vi "VoltageScan_Old.vi"() -> ()   [LabVIEW 2016]
uses:
  <instrlib>/Keithley 24XX/Public/Data/Read (Statistical).vi
  <instrlib>/Keithley 24XX/Public/Data/Read (Single Point).vi
  <instrlib>/Keithley 24XX/Keithley 24XX.lvlib
  <instrlib>/Agilent 428X Series/Agilent 428X Series.lvlib
panel:
  out "error out":errorcluster
  in  "VISA resource name LCR":refnum<visa-resource-name>
  out "Data Status":bool=TRUE
  in  "Open (F:OFF)":bool
  in  "Short (F:OFF)":bool
  out "Primary Value":dbl format="%^.4e"
  out "Secondary Value":dbl format="%^.4e"
  in  "Imp Type (0: CPD)":u32(ring) items=["CPD", "CPQ", "CPG", "CPRP", "CSD", "CSQ", "CSRS", "LPQ", "LPD", "LPG", "LPRP", "LSD", "LSQ", "LSRS", "RX", "ZTD", "ZTR", "GB", "YTD", "YTR"]
  in  "Freq Value (Hz)(1.0 kHz)":dbl=1000.0 min=20.0 max=30000000.0 step=10.0 format="%.4e"
  in  "Voltage Level (V)(1.0V)":dbl=1.0 min=0.0 max=20.0 step=0.1 format="%.4f"
  in  "Measurement type":enum16{"IV", "CV", "Test"}(ring)
  out "Voltage":sgl
  out "Current*Resistance":sgl
  in  "Enable Voltage Auto Range (T:Enable)":bool=TRUE
  in  "Single measurement?":bool=TRUE
  in  "Statistical Operation (0: Mean)":u16(ring) items=["Mean", "Standard Deviation", "Maximum", "Minimum", "Peak to Peak"]
  in  "Sample Count (10)":i32=10
  in  "Source Mode  (0: Voltage)":u16(ring) items=["Voltage", "Current"]
  in  "Compliance  Level (uA)":dbl=0.1
  in  "Voltage":dbl=1.0
  in  "Voltage Manual Range (1.0)":dbl=1.0
  out "Resistance":sgl
  out "Current":sgl
  in  "Serial Configuration":T1={"Baud Rate"=9600, "Parity"=0, "Data Bits"=8, "Stop Bits"=10, "Flow Control"=0} {"Flow Control" items=["None", "XON/XOFF", "RTS/CTS", "XON/XOFF & RTS/CTS", "DTR/DSR", "XON/XOFF & DTR/DSR"]; "Stop Bits" items=["1.0"=10, "1.5"=15, "2.0"=20]; "Data Bits" items=["7"=7, "8"=8]; "Parity" items=["None", "Odd", "Even", "Mark", "Space"]; "Baud Rate" items=["300"=300, "600"=600, "1200"=1200, "2400"=2400, "4800"=4800, "9600"=9600, "19200"=19200]}
  in  "VISA resource name":refnum<visa-resource-name>
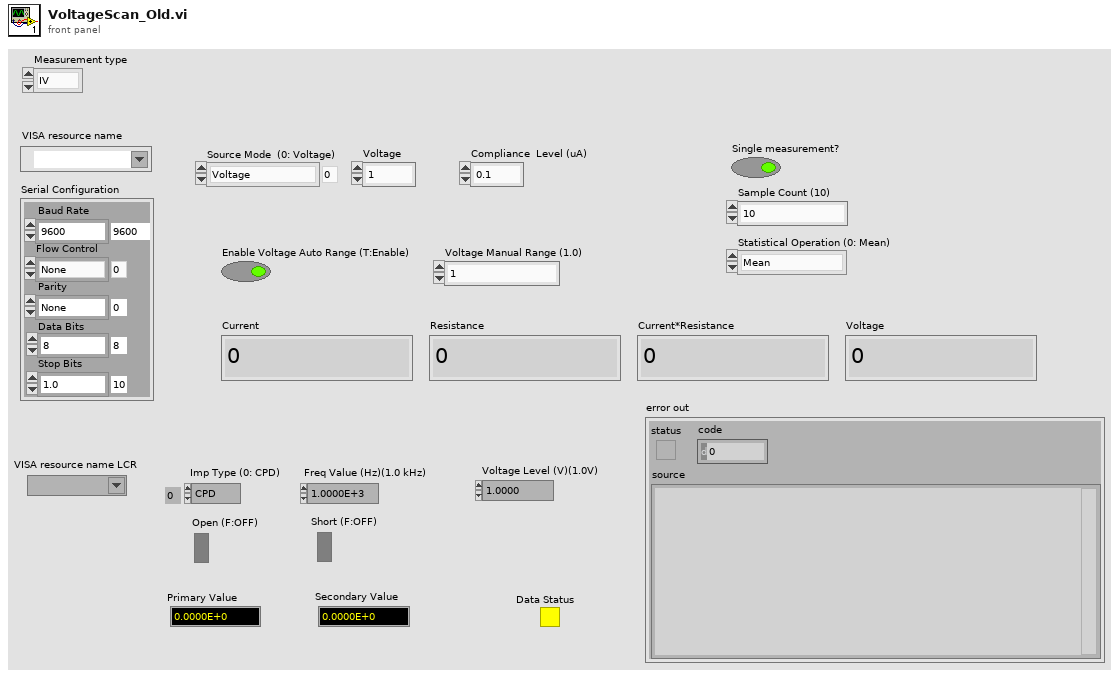
[diagram p1: front panel]
types:
  T1 = cluster{"Baud Rate":u32, "Parity":u16, "Data Bits":u16, "Stop Bits":u16, "Flow Control":u16}
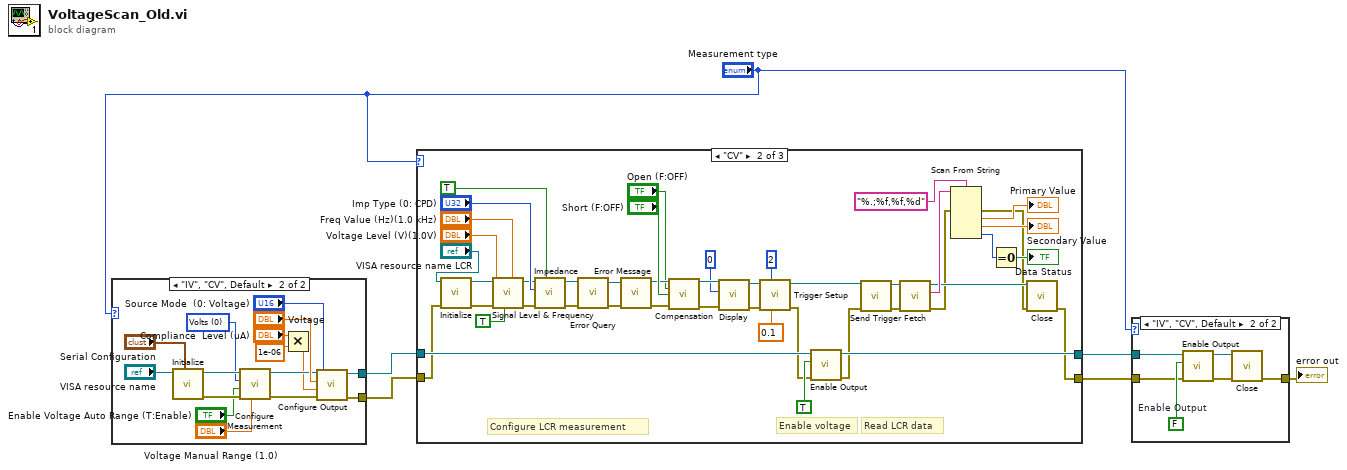
[diagram p0: block diagram]
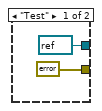
[diagram p3: hidden frame]
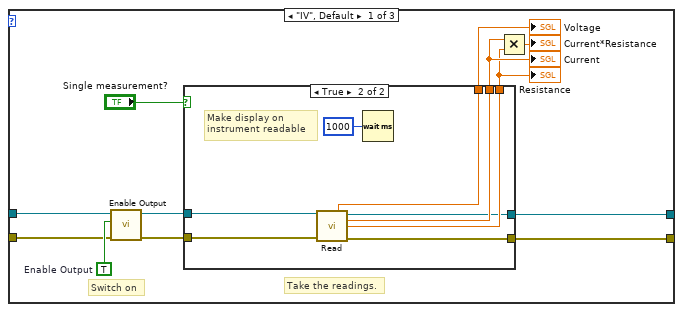
[diagram p4: hidden frame]
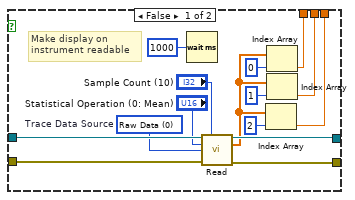
[diagram p5: hidden frame]
diagram:
  n1 = case shown="\"IV\", \"CV\", Default" "Measurement type" {
    tunnel: [errorcluster {"status"=FALSE, "code"=0, "source"=""} ("error out") w10] -> w4
    tunnel: [refnum<visa-resource-name> refnum ("VISA resource name out") w9] -> w3
    frame "Test" {
    }
    frame "IV", "CV", Default {
      w20 = u16 0 items=["Volts", "Current", "Resistance"] ("Function (0: Volts)")
      n2 = call <instrlib>:"Initialize.vi"("Serial Configuration"="Serial Configuration", "VISA resource name"="VISA resource name") -> ("error out"=w21:errorcluster, "VISA resource name out"=w22:refnum<visa-resource-name>)  [unwired: 8 in]
      n3 = call <instrlib>:"Configure Measurement.vi"("Manual Range (1.0)"="Voltage Manual Range (1.0)", "error in (no error)"=w21, "Enable Auto Range (T:Enable)"="Enable Voltage Auto Range (T:Enable)", "Function (0: Volts)"=w20, "VISA resource name"=w22) -> ("error out"=w15:errorcluster, "VISA resource name out"=w16:refnum<visa-resource-name>)  [unwired: 5 in]
      n4 = Multiply(x="Compliance  Level (uA)", y=1e-06) -> (x*y=w12:dbl)
      n5 = call <instrlib>:"Configure Output.vi"("Source Mode  (0: Voltage)"="Source Mode  (0: Voltage)", "error in (no error)"=w15, "Compliance  Level (0.1)"=w12, "Output Level (0)"="Voltage", "VISA resource name"=w16) -> ("error out"=w10:errorcluster, "VISA resource name out"=w9:refnum<visa-resource-name>)  [unwired: 5 in]
    }
  }
  n6 = case shown="\"CV\"" "Measurement type" {
    tunnel: [w36 w63 w104] -> w6
    tunnel: [w35 w101 w105] -> w5
    tunnel: w4 -> [w27 w75 w104]
    tunnel: w3 -> [w28 w102 w105]
    frame "IV", Default {
      w29 = TRUE  # Enable Output
      # "Take the readings."
      # "Switch on"
      n7 = call <instrlib>:"Enable Output.vi"("error in (no error)"=w27, "Enable Output (T: Enable)"=w29, "VISA resource name"=w28) -> ("error out"=w25:errorcluster, "VISA resource name out"=w26:refnum<visa-resource-name>)  [unwired: 7 in]
      n8 = case shown="True" "Single measurement?" {
        tunnel: [w42 w59] -> w32
        tunnel: [w41 w58] -> w31
        tunnel: [w50 w57] -> w36
        tunnel: [w48 w56] -> w35
        tunnel: w25 -> [w51 w55]
        tunnel: w26 -> [w49 w54]
        tunnel: [w38 w53] -> w30
        frame False {
          w43 = u16 0 items=["Raw Data", "Math Data", "Limit Data"]  # Trace Data Source
          # "Make display on instrument readable"
          n9 = Wait (ms)(milliseconds to wait=u32 1000) -> ()  [unwired: 1 out]
          n10 = call-poly <instrlib>:"Read.vi"("VISA resource name"=w49, "Sample Count (2)"="Sample Count (10)", "Statistical Operation (0: Mean)"="Statistical Operation (0: Mean)", "Trace Data Source (0: Raw Data)"=w43, "error in (no error)"=w51) -> ("VISA resource name out"=w48:refnum<visa-resource-name>, "Statistical Operation Results"=w39:dbl[], "error out"=w50:errorcluster)  [unwired: 8 in]
          n11 = Index Array(array=w39, index=2) -> (element=w41:dbl)
          n12 = Index Array(array=w39, index=0) -> (element=w38:dbl)
          n13 = Index Array(array=w39, index=1) -> (element=w42:dbl)
        }
        frame True {
          # "Make display on instrument readable"
          n14 = call-poly <instrlib>:"Read.vi"("VISA resource name"=w54, "error in (no error)"=w55) -> ("Voltage"=w53:sgl, "VISA resource name out"=w56:refnum<visa-resource-name>, "Current"=w59:sgl, "Resistance"=w58:sgl, "error out"=w57:errorcluster)  [unwired: 7 in, 2 out]
          n15 = Wait (ms)(milliseconds to wait=u32 1000) -> ()  [unwired: 1 out]
        }
      }
      "Current" <- w32
      "Resistance" <- w31
      "Voltage" <- w30
      n16 = Multiply(x=w32, y=w31) -> (x*y=→"Current*Resistance":dbl)
    }
    frame "CV" {
      # "Configure LCR measurement"
      # "Read LCR data"
      # "Enable voltage"
      n17 = call <instrlib>:"Initialize.vi"("error in (no error)"=w75, "VISA resource name"="VISA resource name LCR") -> ("error out"=w91:errorcluster, "VISA resource name out"=w90:refnum<visa-resource-name>)  [unwired: 8 in]
      n18 = call <instrlib>:"Signal Level & Frequency.vi"("Frequency Value (Hz) (100KHz)"="Freq Value (Hz)(1.0 kHz)", "Oscillator Select (T: Voltage)"=TRUE, "error in (no error)"=w91, "Voltage Level (V) (5mV)"="Voltage Level (V)(1.0V)", "VISA resource name"=w90) -> ("error out"=w78:errorcluster, "VISA resource name out"=w77:refnum<visa-resource-name>)  [unwired: 5 in]
      n19 = call <instrlib>:"Impedance.vi"("Auto Range (F: Off)"=TRUE ("Auto Range (On:T)"), "error in (no error)"=w78, "Imp Type (0: CPD)"="Imp Type (0: CPD)", "VISA resource name"=w77) -> ("error out"=w84:errorcluster, "VISA resource name out"=w85:refnum<visa-resource-name>)  [unwired: 6 in]
      n20 = call <instrlib>:"Error Query.vi"("error in (no error)"=w84, "VISA resource name"=w85) -> ("error out"=w92:errorcluster, "VISA resource name out"=w86:refnum<visa-resource-name>)  [unwired: 6 in, 2 out]
      n21 = call <instrlib>:"Error Message.vi"("error in (no error)"=w92, "VISA resource name"=w86) -> ("error out"=w87:errorcluster, "VISA resource name out"=w88:refnum<visa-resource-name>)  [unwired: 5 in, 3 out]
      n22 = call <instrlib>:"Compensation.VI"("VISA resource name"=w88, "OPEN (F:OFF)"="Open (F:OFF)", "SHORT (F:OFF)"="Short (F:OFF)", "error in (no error)"=w87) -> ("VISA resource name out"=w99:refnum<visa-resource-name>, "error out"=w98:errorcluster)  [unwired: 10 in]
      n23 = call <instrlib>:"Display.vi"("error in (no error)"=w98, "Display Page (0: Measurement)"=u32 0 ("Display Page (Measurment:0)"), "VISA resource name"=w99) -> ("error out"=w96:errorcluster, "VISA resource name out"=w97:refnum<visa-resource-name>)  [unwired: 7 in]
      n24 = call <instrlib>:"Trigger Setup.vi"("Delay Value (s) (0.0)"=0.1, "Trigger Source (0: Internal)"=u32 2 ("bus triggering"), "error in (no error)"=w96, "VISA resource name"=w97) -> ("error out"=w74:errorcluster, "VISA resource name out"=w64:refnum<visa-resource-name>)  [unwired: 6 in]
      n25 = call <instrlib>:"Enable Output.vi"("error in (no error)"=w74, "Enable Output (T: Enable)"=TRUE ("Enable Output"), "VISA resource name"=w102) -> ("error out"=w62:errorcluster, "VISA resource name out"=w101:refnum<visa-resource-name>)  [unwired: 7 in]
      n26 = call <instrlib>:"Send Trigger.vi"("error in (no error)"=w62, "VISA resource name"=w64) -> ("error out"=w66:errorcluster, "VISA resource name out"=w71:refnum<visa-resource-name>)  [unwired: 8 in]
      n27 = call <instrlib>:"Fetch.vi"("error in (no error)"=w66, "VISA resource name"=w71) -> ("error out"=w61:errorcluster, "Returned Data"=w70:string, "VISA resource name out"=w65:refnum<visa-resource-name>)  [unwired: 7 in]
      n28 = Scan From String(format string="%.;%f,%f,%d", input string=w70, error in=w61) -> (error out=w60:errorcluster, output 1=→"Primary Value":dbl, output 2=→"Secondary Value":dbl, output 3=w67:i32)  [unwired: 4 in, 2 out]
      n29 = Equal To 0?(x=w67) -> (x = 0?=→"Data Status":bool)
      n30 = call <instrlib>:"Close.vi"("error in (no error)"=w60, "VISA resource name"=w65) -> ("error out"=w63:errorcluster)  [unwired: 9 in]
    }
    frame "Test" {
    }
  }
  n31 = case shown="\"IV\", \"CV\", Default" "Measurement type" {
    tunnel: w6 -> [w106 w109]
    tunnel: w5 -> [_ w108]
    tunnel: [w106 w107] -> w1
    frame "Test" {
    }
    frame "IV", "CV", Default {
      w112 = FALSE  # Enable Output
      n32 = call <instrlib>:"Enable Output.vi"("error in (no error)"=w109, "Enable Output (T: Enable)"=w112, "VISA resource name"=w108) -> ("error out"=w110:errorcluster, "VISA resource name out"=w111:refnum<visa-resource-name>)  [unwired: 7 in]
      n33 = call <instrlib>:"Close.vi"("error in (no error)"=w110, "VISA resource name"=w111) -> ("error out"=w107:errorcluster)  [unwired: 9 in]
    }
  }
  "error out" <- w1
